vi "Carmera Motor Buttons.vi"(8 "error in (no error)":errorcluster, 10 "Buttons":bool[](array[boolean])) -> (0 "error out":errorcluster)   [LabVIEW 2014]
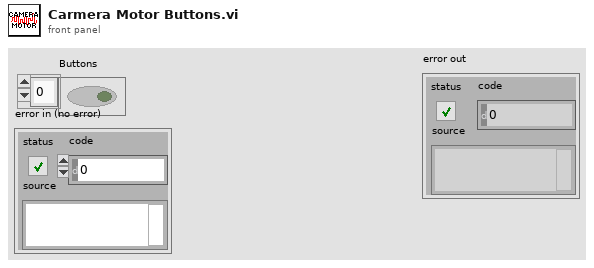
[diagram p1: front panel]
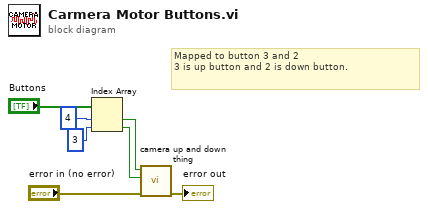
[diagram p0: block diagram]
diagram:
  # "Mapped to button 3 and 2\n3 is up button and 2 is down button."
  n1 = Index Array(array="Buttons", index #1=4 ("index"), index #2=3 ("index")) -> (element #1=w4:bool, element #2=w3:bool)
  n2 = call "camera up and down thing.vi"("error in (no error)"="error in (no error)", "down button"=w3, "up button"=w4) -> ("error out"=→"error out":errorcluster)  [unwired: 8 in]
